vi "Resize UI Elements.vi"(8 "error in (no error)":errorcluster, 10 "New Tab dimensions":T1, 11 "Report Viewer in":refnum<class "Report Viewer.lvclass">) -> (0 "error out":errorcluster, 3 "Report Viewer out":refnum<class "Report Viewer.lvclass">)   [LabVIEW 2019, in "Report Viewer.lvlib" / "Report Viewer.lvclass"]
uses:
  Library/Report Viewer.lvclass
  <vilib>/Utility/miscctls.llb/LVBoundsTypeDef.ctl
  Library/Report Viewer.lvclass/Report Viewer.ctl
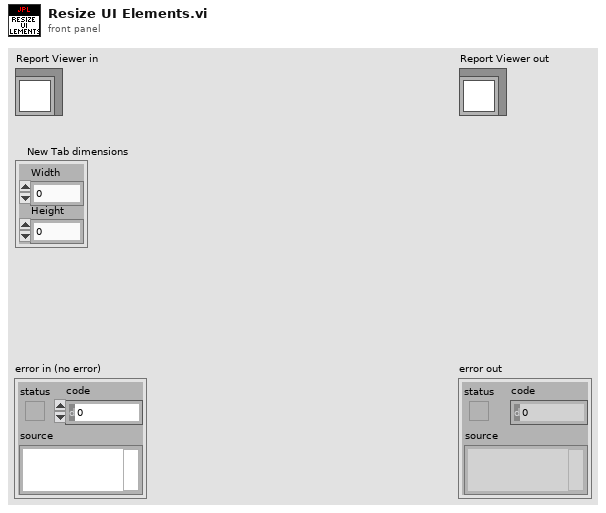
[diagram p1: front panel]
types:
  T1 = typedef "LVBoundsTypeDef.ctl" = cluster{"Width":u32, "Height":u32}
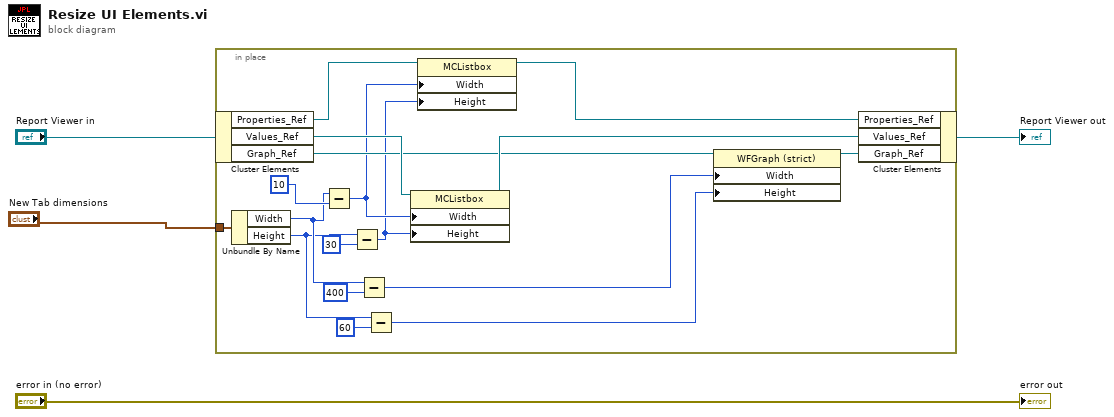
[diagram p0: block diagram]
diagram:
  n1 = in-place {
    in-place-border: "New Tab dimensions" -> [w20]
    n2 = in-place-cluster #1("Report Viewer in") -> ("Properties_Ref"=w18:refnum<vi>, "Values_Ref"=w21:refnum<vi>, "Graph_Ref"=w16:refnum<vi>)
    n3 = Unbundle By Name(w20) -> ("Width"=w11:u32, "Height"=w10:u32)
    n4 = Subtract(x=w11, y=10) -> (x-y=w14:u32)
    n5 = Subtract(x=w10, y=u32 30) -> (x-y=w13:u32)
    n6 = Subtract(x=w11, y=u32 400) -> (x-y=w7:u32)
    n7 = Subtract(x=w10, y=u32 60) -> (x-y=w8:u32)
    n8 = property class="MCListbox"(reference=w21, "Width"=w14, "Height"=w13) -> (reference out=w19:refnum<vi>)  [unwired: 1 in, 1 out]
    n9 = property class="MCListbox"(reference=w18, "Width"=w14, "Height"=w13) -> (reference out=w17:refnum<vi>)  [unwired: 1 in, 1 out]
    n10 = property class="WFGraph (strict)"(reference=w16, "Width"=w7, "Height"=w8) -> (reference out=w15:refnum<vi>)  [unwired: 1 in, 1 out]
    n11 = in-place-cluster #1("Properties_Ref"=w17, "Values_Ref"=w19, "Graph_Ref"=w15) -> (→"Report Viewer out":refnum<class "Report Viewer.lvclass">)
  }
  "error out" <- "error in (no error)"
